vi "BMark_Get Bookmarks.vi"(8 "error in (no error)":errorcluster, 11 "App Info":T1) -> (0 "error out":errorcluster, 2 "possible undisplayed bookmarks":bool, 3 "bookmarks":T2[](array[typedef]))   [LabVIEW 2017]
uses:
  controls/BMark_Bookmark Data.ctl
  controls/BMark_VI_Identifier.ctl
  <vilib>/addons/analyzer/_analyzerctrls.llb/VIAnCtl Analysis App Info.ctl
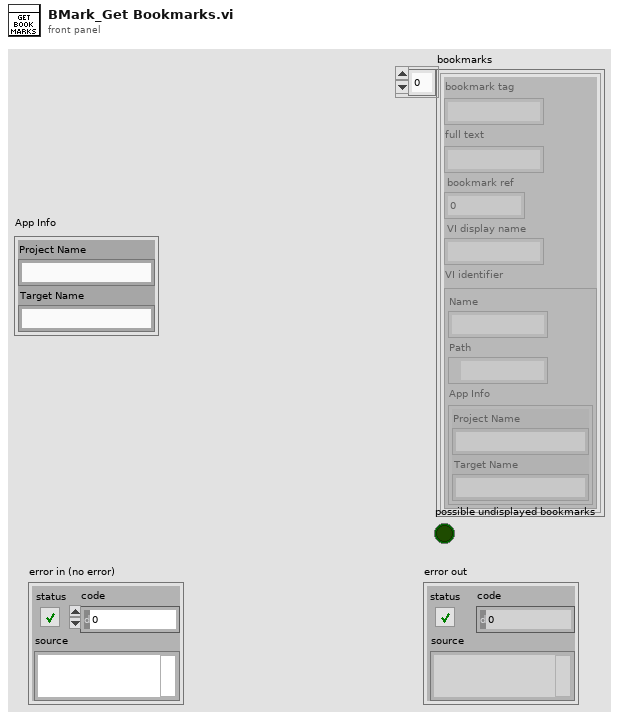
[diagram p1: front panel]
types:
  T1 = typedef "VIAnCtl Analysis App Info.ctl" = cluster{"Project Name":string, "Target Name":string}
  T2 = typedef "BMark_Bookmark Data.ctl" = cluster{"bookmark tag":string, "full text":string, "bookmark ref":i32, "VI display name":string, "VI identifier":T3}
  T3 = typedef "BMark_VI_Identifier.ctl" = cluster{"Name":string, "Path":path, "App Info":T1}
  T4 = typedef "BMark_Array of Bookmarks.ctl" = T5[]
  T5 = typedef "BMark_Bookmark Cluster.ctl" = cluster{"bookmark ref":i32, "bookmark":string, "label text":string, "VI identifier":T3}
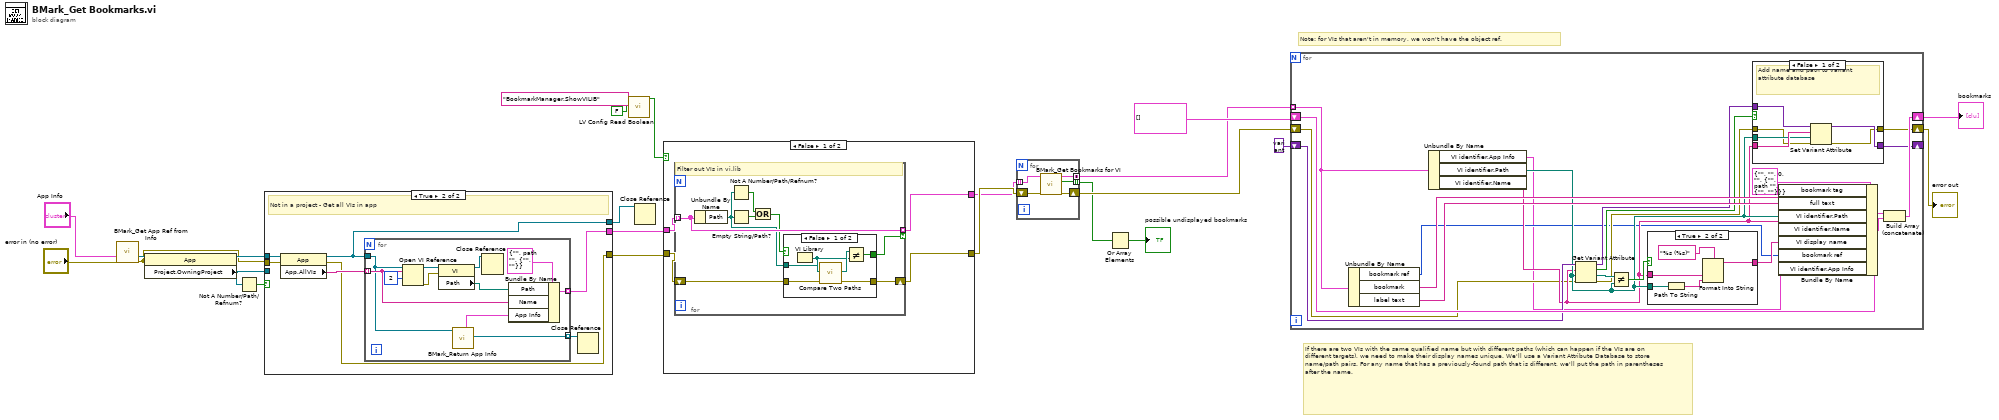
[diagram p0: block diagram]
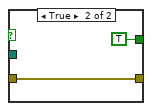
[diagram p2: hidden frame]
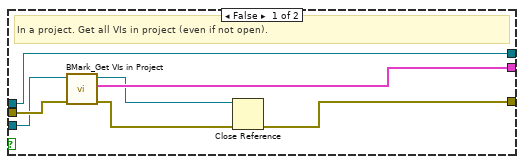
[diagram p4: hidden frame]
diagram:
  # "Note: for VIs that aren't in memory, we won't have the object ref."
  # "If there are two VIs with the same qualified name but with different paths (which can happen if the VIs are on different targets), we need to make their display names unique. We'll use a Variant Attribute Database to store name/path pairs. For any name that has a previously-found path that is different, we'll put the path in parentheses after the name."
  n1 = call "BMark_Get App Ref from Info.vi"("error in (no error)"="error in (no error)", "Analysis App Info"="App Info") -> ("error out"=w2:errorcluster, "Analysis App ref"=w4:refnum<vi>)  [unwired: 8 in]
  n2 = property class="App"(reference=w4, error in=w2) -> (reference out=w20:refnum<vi>, "Project.OwningProject"=w19:refnum<vi>)  [unwired: 1 out]
  n3 = Not A Number/Path/Refnum?(number/path/refnum=w19) -> (NaN/Path/Refnum?=w21:bool)
  n4 = case shown="True" w21 {
    tunnel: w20 -> [w28 w37]
    tunnel: w19 -> [w26 _]
    tunnel: [w24 w33] -> w15
    tunnel: w2 -> [w30 w36]
    tunnel: [w29 w34] -> w10
    tunnel: [w28 w32] -> w1
    frame False {
      # "In a project. Get all VIs in project (even if not open)."
      n5 = call "BMark_Get VIs in Project.vi"("error in (no error)"=w30, "project"=w26) -> ("error out"=w27:errorcluster, "Array of VIs"=w29:T3[], "project out"=w25:refnum<vi>)  [unwired: 7 in]
      n6 = Close Reference(reference=w25, error in (no error)=w27) -> (error out=w24:errorcluster)
    }
    frame True {
      # "Not in a project - Get all VIs in app"
      n7 = property class="App"(reference=w37, error in=w36) -> (reference out=w32:refnum<vi>, error out=w33:errorcluster, "App.AllVIs"=w35:string[])
      n8 = for {
        tunnel: w35 -> [w43] mode=indexing
        tunnel: [w47] -> w34 mode=indexing
        tunnel: w32 -> [w42]
        tunnel: [w39] -> w31 mode=indexing
        n9 = Open VI Reference(application reference (local)=w42, vi path=w43, options=2) -> (vi reference=w46:refnum<vi>, error out=w45:errorcluster)  [unwired: 3 in]
        n10 = property class="VI"(reference=w46, error in=w45) -> (reference out=w40:refnum<vi>, "Path"=w44:path)  [unwired: 1 out]
        n11 = call "BMark_Return App Info.vi"("App Refnum in"=w42) -> ("App Refnum for Opening VI"=w39:refnum<vi>, "App Info"=w41:T1)  [unwired: 8 in, 1 out]
        n12 = Close Reference(reference=w40) -> ()  [unwired: 1 in, 1 out]
        n13 = Bundle By Name(cluster=T3 {"Name"="", "Path"=path "", "App Info"={"Project Name"="", "Target Name"=""}} ("Cluster"), "Path"=w44, "Name"=w43, "App Info"=w41) -> (w47:T3)
      }
      n14 = Close Reference(reference=w31) -> ()  [unwired: 1 in, 1 out]
    }
  }
  n15 = call <resource>:"LV Config Read Boolean.vi"("default value"=FALSE, "key"="BookmarkManager.ShowVILIB") -> ("value"=w11:bool)  [unwired: 3 in, 2 out]
  n16 = Close Reference(reference=w1) -> ()  [unwired: 1 in, 1 out]
  n17 = case shown="False" w11 {
    tunnel: w15 -> [w52 w70]
    tunnel: [w50 w70] -> w14
    tunnel: w10 -> [w51 w69]
    tunnel: [w49 w69] -> w9
    frame False {
      n18 = for {
        shift-right: [w59] -> w50
        shift-left: w52 -> [w60]
        tunnel: w51 -> [w57] mode=indexing
        tunnel: [w57] -> w49 mode=indexing if=w58
        # "Filter out VIs in vi.lib"
        n19 = Unbundle By Name(w57) -> ("Path"=w56:path)
        n20 = Not A Number/Path/Refnum?(number/path/refnum=w56) -> (NaN/Path/Refnum?=w55:bool)
        n21 = Empty String/Path?(string/path=w56) -> (empty?=w54:bool)
        n22 = Or(x=w55, y=w54) -> (x .or. y?=w53:bool)
        n23 = case shown="False" w53 {
          tunnel: w60 -> [w64 w67]
          tunnel: [w63 w67] -> w59
          tunnel: w56 -> [w62 _]
          tunnel: [w61 TRUE] -> w58
          frame False {
            n24 = VI Library() -> (path=w65:path)
            n25 = call <vilib>:"Compare Two Paths.vi"("error in (no error)"=w64, "Path 2"=w65, "Path 1"=w62) -> ("error out"=w63:errorcluster, "Common Path"=w66:path)  [unwired: 5 in, 2 out]
            n26 = Not Equal?(x=w66, y=w65) -> (x != y?=w61:bool)
          }
          frame True {
          }
        }
      }
    }
    frame True {
    }
  }
  n27 = for {
    shift-right: [w74] -> w17
    shift-left: w14 -> [w75]
    tunnel: [w73] -> w18 mode=concatenating
    tunnel: w9 -> [w72] mode=indexing
    tunnel: [w71] -> w7 mode=indexing
    n28 = call "BMark_Get Bookmarks for VI.vi"("error in (no error)"=w75, "VI"=w72) -> ("error out"=w74:errorcluster, "possible undisplayed bookmarks"=w71:bool, "Array of bookmarks"=w73:T4)  [unwired: 7 in]
  }
  n29 = Or Array Elements(Boolean array=w7) -> (logical OR=→"possible undisplayed bookmarks":bool)
  n30 = for {
    shift-right: [w95] -> w22
    shift-left: T2[] [] -> [w96]
    tunnel: w18 -> [w81] mode=indexing
    shift-right: [w82] -> w16
    shift-left: w17 -> [w78]
    shift-right: [w90] -> _
    shift-left: variant -> [w89]
    n31 = Unbundle By Name(w81) -> ("bookmark ref"=w77:i32, "bookmark"=w91:string, "label text"=w92:string)
    n32 = Unbundle By Name(w81) -> ("VI identifier.App Info"=w76:T1, "VI identifier.Path"=w80:path, "VI identifier.Name"=w79:string)
    n33 = Get Variant Attribute(Variant=w89, name=w79, default value (empty Variant)=w80, error in=w78) -> (duplicate Variant=w85:variant, found=w84:bool, value=w88:path, error out=w83:errorcluster)
    n34 = Not Equal?(x=w88, y=w80) -> (x != y?=w86:bool)
    n35 = case shown="True" w86 {
      tunnel: w80 -> [_ w108]
      tunnel: w79 -> [w105 w107]
      tunnel: [w105 w106] -> w87
      frame False {
      }
      frame True {
        n36 = Path To String(path=w108) -> (string=w109:string)
        n37 = Format Into String(format string="%s (%s)", w107, w109) -> (resulting string=w106:string)  [unwired: 2 in, 1 out]
      }
    }
    n38 = case shown="False" w84 {
      tunnel: [w102 w104] -> w90
      tunnel: w85 -> [w101 w104]
      tunnel: w79 -> [w100 _]
      tunnel: w80 -> [w99 _]
      tunnel: w83 -> [w98 w103]
      tunnel: [w97 w103] -> w82
      frame False {
        # "Add name and path to variant attribute database"
        n39 = Set Variant Attribute(Variant=w101, name=w100, value=w99, error in=w98) -> (Variant out=w102:variant, error out=w97:errorcluster)  [unwired: 1 out]
      }
      frame True {
      }
    }
    n40 = Bundle By Name(cluster=T2 {"bookmark tag"="", "full text"="", "bookmark ref"=0, "VI display name"="", "VI identifier"={"Name"="", "Path"=path "", "App Info"={"Project Name"="", "Target Name"=""}}} ("bookmark item"), "bookmark tag"=w91, "full text"=w92, "VI identifier.Path"=w80, "VI identifier.Name"=w79, "VI display name"=w87, "bookmark ref"=w77, "VI identifier.App Info"=w76) -> (w93:T2)
    n41 = Build Array (concatenate)(w96, w93) -> (w95:T2[])
  }
  "bookmarks" <- w22
  "error out" <- w16
